vi "Set Sweep Timeout.vi"(0 "VISA resource name":refnum<visa-resource-name>, 1 "Set Timeout For (0: Sweep Timeout)":u16(ring) items=["Sweep Timeout", "Ordinary Timeout"], 11 "error in (no error)":errorcluster) -> (4 "VISA resource name out":refnum<visa-resource-name>, 15 "error out":errorcluster)   [LabVIEW 2021, in "Keithley 648X Series.lvlib"]
doc: "This private VI works in tandem with <b>Calculate Sweep Timeout</b> to control the VISA timeout settings. This is necessary due to the instrument not responding to queries in a timely manner when performing a voltage sweep."
uses:
  <instrlib>/Keithley 648X Series/Keithley 648X Series.lvlib
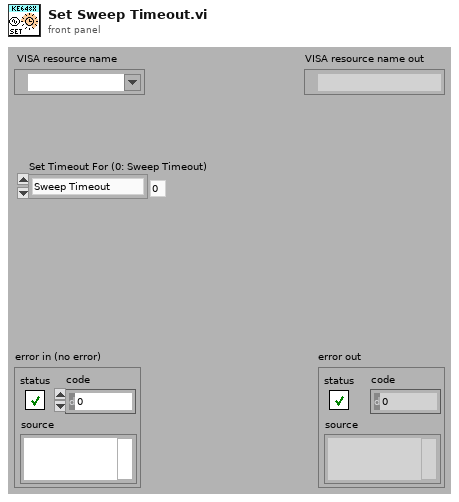
[diagram p1: front panel]
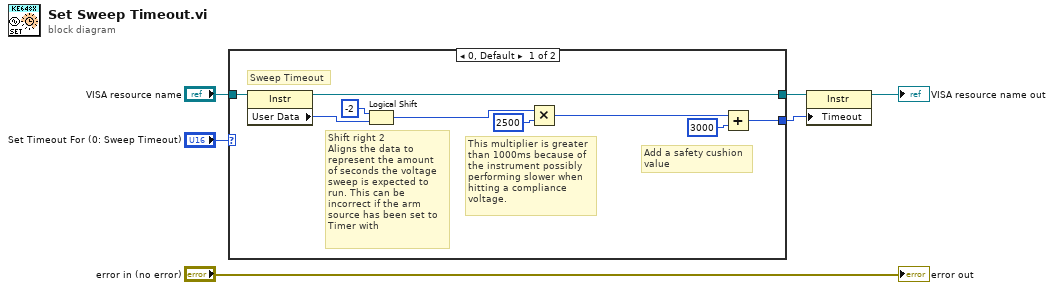
[diagram p0: block diagram]
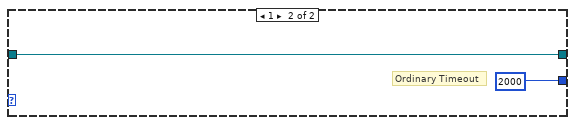
[diagram p2: hidden frame]
diagram:
  n1 = case shown="0, Default" "Set Timeout For (0: Sweep Timeout)" {
    tunnel: [w11 u32 2000 ("General Settings:Timeout Value")] -> w1
    tunnel: "VISA resource name" -> [w15 w16]
    tunnel: [w10 w16] -> w2
    frame 0, Default {
      # "This multiplier is greater\nthan 1000ms because of\nthe instrument possibly\nperforming slower when\nhitting a compliance\nvoltage."
      # "Add a safety cushion\nvalue"
      # "Shift right 2\nAligns the data to \nrepresent the amount\nof seconds the voltage \nsweep is expected to \nrun. This can be \nincorrect if the arm\nsource has been set to\nTimer with"
      # "Sweep Timeout"
      n2 = property class="Instr"(reference=w15) -> (reference out=w10:refnum<visa-resource-name>, "User Data"=w14:u32)  [unwired: 1 in, 1 out]
      n3 = Logical Shift(y=i16 -2, x=w14) -> (x << y=w9:u32)
      n4 = Multiply(x=w9, y=u32 2500) -> (x*y=w7:u32)
      n5 = Add(x=w7, y=u32 3000) -> (x+y=w11:u32)
    }
    frame 1 {
      # "Ordinary Timeout"
    }
  }
  n6 = property class="Instr"(reference=w2, "Timeout"=w1) -> (reference out=→"VISA resource name out":refnum<visa-resource-name>)  [unwired: 1 in, 1 out]
  "error out" <- "error in (no error)"
